vi "Sync.vi"(5 "Username":string, 6 "Password":string, 7 "Address":string, 8 "Error In":errorcluster) -> (0 "Error Out":errorcluster)   [LabVIEW 2018, in "Tests.lvlib" / "SFTP File.lvlib"]
uses:
  SFTP File.lvlib
  src/Toolkit/SFTP File/Support/Open from SFTP.vi
  src/Toolkit/SFTP File/Support/Close to SFTP.vi
  <vilib>/addons/_JKI Toolkits/Caraya/classes/Test/Test.lvclass
  <vilib>/addons/_JKI Toolkits/Caraya/classes/Assert/Assert.lvclass
  src/Toolkit/SFTP File/SFTP File.lvclass
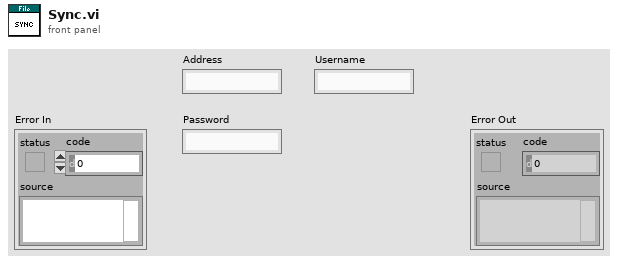
[diagram p1: front panel]
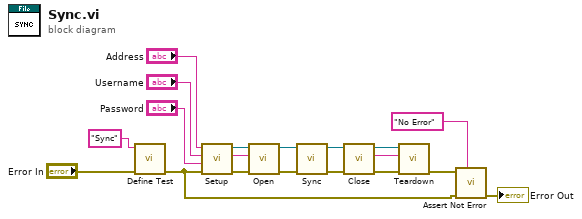
[diagram p0: block diagram]
diagram:
  n1 = call <vilib>:"Define Test.vi"("error in (no error)"="Error In", "Label (VI Title)"="Sync") -> ("error out"=w13:errorcluster)  [unwired: 9 in]
  n2 = call "Setup.vi"("Error In"=w13, "Password"="Password", "Username"="Username", "Address"="Address") -> ("Error Out"=w10:errorcluster, "Temporary File"=w4:string, "SFTP"=w11:refnum<class "SFTP.lvclass">)  [unwired: 5 in]
  n3 = call-poly "Open.vi"("Error In"=w10, "Remote Path"=w4, "SFTP"=w11) -> ("Error Out"=w7:errorcluster, "SFTP File"=w9:refnum<class "SFTP File.lvclass">)  [unwired: 7 in]
  n4 = call "Sync.vi"("Error In"=w7, "SFTP File In"=w9) -> ("Error Out"=w6:errorcluster, "SFTP File Out"=w8:refnum<class "SFTP File.lvclass">)  [unwired: 8 in]
  n5 = call-poly "Close.vi"("Error In"=w6, "SFTP File"=w8) -> ("Error Out"=w3:errorcluster, "Remote Path"=w2:string, "SFTP"=w1:refnum<class "SFTP.lvclass">)  [unwired: 7 in]
  n6 = call "Teardown.vi"("Error In"=w3, "Temporary File"=w2, "SFTP"=w1) -> ("Error Out"=w12:errorcluster)  [unwired: 8 in]
  n7 = call <vilib>:"Assert Not Error.vi"("Label"="No Error", "error in (no error)"=w13, "Not Error?"=w12) -> ("error out"=→"Error Out":errorcluster)  [unwired: 8 in]
